vi "PH_Sound.PlayWaveform.vi"(0 "i ref in":refnum<vi>, 2 "path":path, 5 "error in (no error)":errorcluster) -> (14 "i ref out":refnum<vi>, 19 "error out":errorcluster)   [LabVIEW 2014, in "PH_Sound.lvlib"]
doc: "This VI play a .waf file."
uses:
  PH_Sound.lvlib
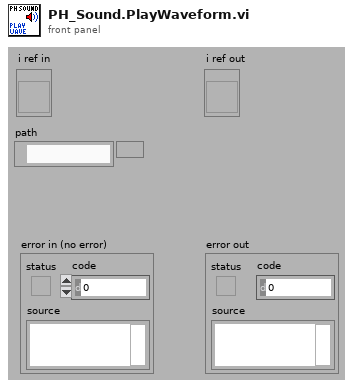
[diagram p1: front panel]
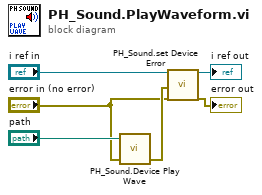
[diagram p0: block diagram]
diagram:
  n1 = call "PH_Sound.Device Play Wave.vi"("error in (no error)"="error in (no error)", "path"="path") -> ("Device error out"=w4:errorcluster)  [unwired: 3 in]
  n2 = call "PH_Sound.set Device Error.vi"("VI in"="i ref in", "Device error"=w4, "error in"="error in (no error)") -> ("VI out"=→"i ref out":refnum<vi>, "error out"=→"error out":errorcluster)  [unwired: 15 in]
